vi "test222.vi"() -> ()   [LabVIEW 2012]
uses:
  <vilib>/Analysis/Matrix/Numeric/Conversions/Array To Matrix - RA2.vi
  <vilib>/Analysis/baseanly.llb/Real Inverse Matrix.vi
  <vilib>/Analysis/_algsub.llb/Real Matrix Trace.vi
  <vilib>/Analysis/Matrix/NI_Matrix.lvlib
  <vilib>/Analysis/NI_AALBase.lvlib
  <vilib>/Analysis/NI_AALPro.lvlib
panel:
  out "Numeric Control":i32
  out "trace":dbl format="%.2f"
  out "millisecond timer value":u32
  out "x-y":u32
  out "x/y":dbl
  out "number of columns":i32
  out "number of rows":i32
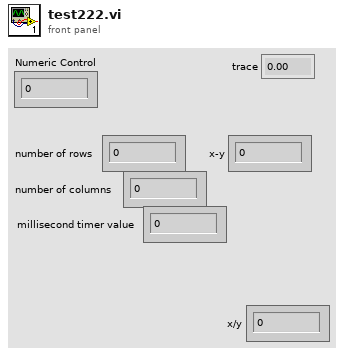
[diagram p1: front panel]
types:
  T1 = typedef "NI_Matrix.lvlib/RealMatrix.ctl" = dbl[][]
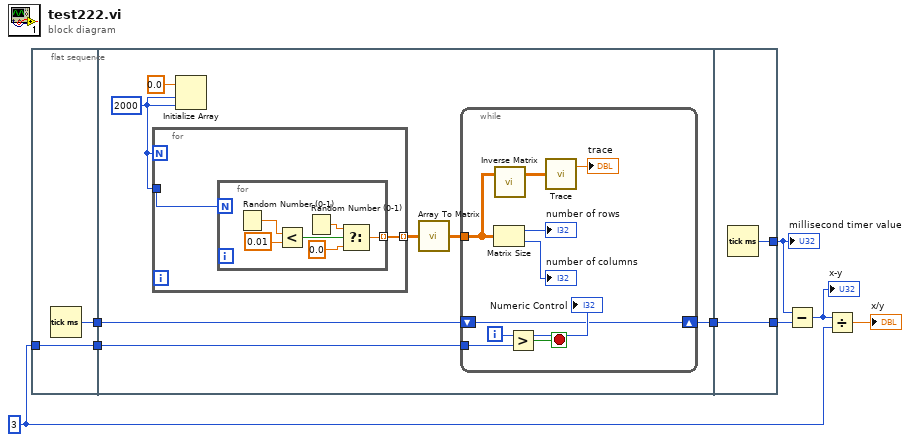
[diagram p0: block diagram]
diagram:
  w6 = 3 ("y")
  n1 = flat-sequence {
    tunnel: w6 -> [w10]
    tunnel: [w10] -> w2
    tunnel: [w9] -> w1
    tunnel: [w17] -> w4
    tunnel: w2 -> [w16]
    tunnel: w1 -> [w15]
    tunnel: [w36] -> w8
    tunnel: w4 -> [w36]
    tunnel: [w35] -> w3
    frame #0 {
      n2 = Tick Count (ms)() -> (millisecond timer value=w9:u32)
    }
    frame #1 {
      w14 = 2000 ("dimension size")
      n3 = for {
        N: w14 -> [_]
        tunnel: [w19] -> w12 mode=indexing
        tunnel: w14 -> [w18]
        n4 = for {
          N: w18 -> [_]
          tunnel: [w20] -> w19 mode=indexing
          n5 = Random Number (0-1)() -> (number: 0 to 1=w25:dbl)
          n6 = Less?(x=w25, y=0.01) -> (x < y?=w23:bool)
          n7 = Random Number (0-1)() -> (number: 0 to 1=w22:dbl)
          n8 = Select(t=w22, s=w23, f=0.0) -> (s? t:f=w20:dbl)
        }
      }
      n9 = Initialize Array(0.0 ("element"), w14, w14) -> ()  [unwired: 1 out]
      n10 = call-poly <vilib>:"Array To Matrix.vi"("Real 2D Array"=w12) -> ("Real Matrix"=w11:T1)
      n11 = while {
        shift-right: [w30] -> w17
        shift-left: w15 -> [w30]
        tunnel: w16 -> [w29]
        tunnel: w11 -> [w26]
        i -> [w32]
        stop <- w31 stop-if-true
        n12 = Matrix Size(0:w26) -> (1:→"number of rows":i32, 2:→"number of columns":i32)
        n13 = call-poly <vilib>:"Inverse Matrix.vi"("Input Matrix"=w26) -> ("Inverse Matrix"=w27:T1)  [unwired: 1 in, 1 out]
        n14 = Greater?(x=w32, y=w29) -> (0:w31:bool)
        n15 = call-poly <vilib>:"Trace.vi"("Input Matrix"=w27) -> ("trace"=→"trace":dbl)  [unwired: 1 out]
        "Numeric Control" <- w32
      }
    }
    frame #2 {
      n16 = Tick Count (ms)() -> (millisecond timer value=w35:u32)
    }
  }
  n17 = Subtract(x=w3, y=w8) -> (x-y=w7:u32)
  "x-y" <- w7
  n18 = Divide(x=w7, y=w6) -> (x/y=→"x/y":dbl)
  "millisecond timer value" <- w3
